vi "Area of Triangle D4.vi"(9 "Side C (cm)":dbl, 10 "Side B(cm)":dbl, 11 "Side A (cm)":dbl) -> (3 "Area Of Triangle":dbl)   [LabVIEW 2026]
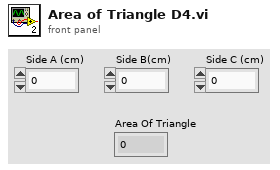
[diagram p1: front panel]
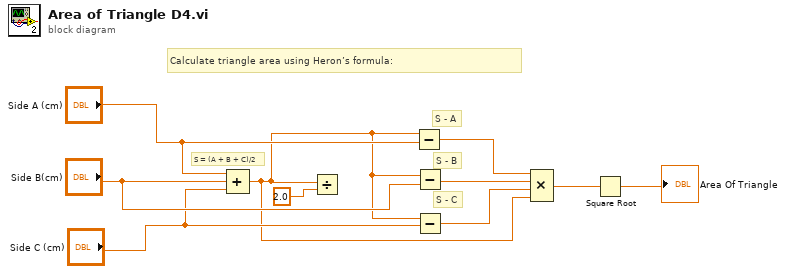
[diagram p0: block diagram]
diagram:
  # "Calculate triangle area using Heron’s formula:"
  # "S - C"
  # "S - B"
  # "S - A"
  # "S = (A + B + C)/2"
  n1 = Compound Arithmetic op=ADD("Side A (cm)", "Side B(cm)", "Side C (cm)") -> (w4:dbl)
  n2 = Divide(x=w4, y=2.0) -> ()  [unwired: 1 out]
  n3 = Subtract(x=w4, y="Side A (cm)") -> (x-y=w7:dbl)
  n4 = Subtract(x=w4, y="Side B(cm)") -> (x-y=w6:dbl)
  n5 = Subtract(x=w4, y="Side C (cm)") -> (x-y=w5:dbl)
  n6 = Compound Arithmetic op=MULTIPLY(w7, w6, w5, w4) -> (w3:dbl)
  n7 = Square Root(x=w3) -> (sqrt(x)=→"Area Of Triangle":dbl)
